vi "Tree Sync_Sync Top Item.vi"(8 "error in":errorcluster, 10 "Changed Tree Control Ref":refnum<vi>, 11 "All Tree Control Refs":refnum<vi>[](array[refnum])) -> (0 "error out":errorcluster)   [LabVIEW 2023]
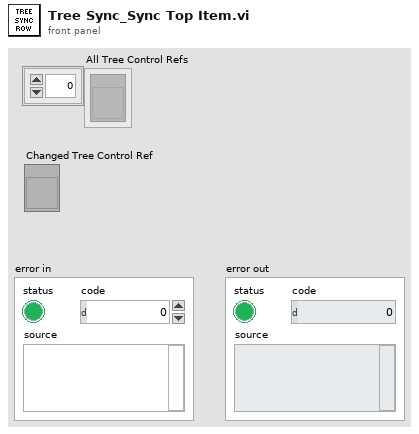
[diagram p1: front panel]
types:
  T1 = typedef "LVNodeAndColumnTypeDef.ctl" = cluster{"Node":string, "Column":i32}
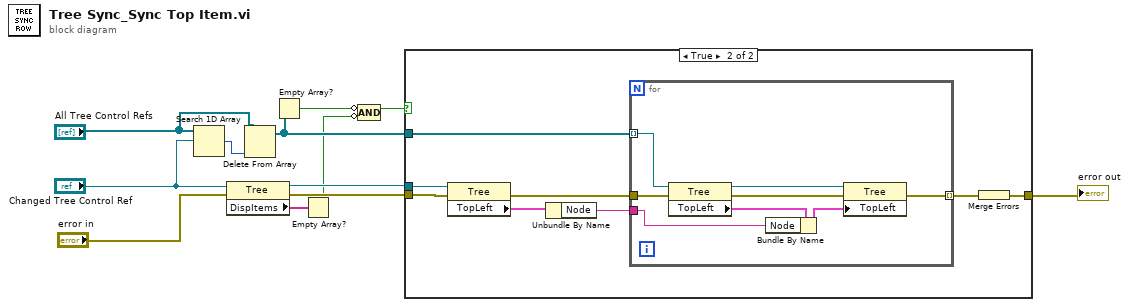
[diagram p0: block diagram]
diagram:
  n1 = Search 1D Array(1D array="All Tree Control Refs", element="Changed Tree Control Ref") -> (index of element=w11:i32)  [unwired: 1 in]
  n2 = property class="Tree"(reference="Changed Tree Control Ref", error in="error in") -> (reference out=w7:refnum<vi>, error out=w5:errorcluster, "DispItems"=w4:string[])
  n3 = Delete From Array(array="All Tree Control Refs", index=w11) -> (array with subset deleted=w9:refnum<vi>[])  [unwired: 1 in, 1 out]
  n4 = Empty Array?(array=w9) -> (empty?=w3:bool)
  n5 = Empty Array?(array=w4) -> (empty?=w2:bool)
  n6 = Compound Arithmetic op=AND(invert w3, invert w2) -> (w1:bool)
  n7 = case shown="True" w1 {
    tunnel: w9 -> [_ w21]
    tunnel: [w13 w19] -> w10
    tunnel: w7 -> [_ w17]
    tunnel: w5 -> [w13 w14]
    frame False {
    }
    frame True {
      n8 = property class="Tree"(reference=w17, error in=w14) -> (error out=w16:errorcluster, "TopLeft"=w18:T1)  [unwired: 1 out]
      n9 = Unbundle By Name(w18) -> ("Node"=w15:string)
      n10 = for {
        tunnel: w21 -> [w29] mode=indexing
        tunnel: w15 -> [w25]
        tunnel: w16 -> [w22]
        tunnel: [w23] -> w20 mode=indexing
        n11 = property class="Tree"(reference=w29, error in=w22) -> (reference out=w28:refnum<vi>, error out=w24:errorcluster, "TopLeft"=w27:T1)
        n12 = Bundle By Name(cluster=w27, "Node"=w25) -> (w26:T1)
        n13 = property class="Tree"(reference=w28, error in=w24, "TopLeft"=w26) -> (error out=w23:errorcluster)  [unwired: 1 out]
      }
      n14 = Merge Errors(w20) -> (w19:errorcluster)
    }
  }
  "error out" <- w10
